vi "Convert to GEV Mono12Packed.vi"(10 "Source Image In":u8[](array[numeric])) -> (2 "Source Image Out":u8[](array[numeric]))   [LabVIEW 2021, in "DecodetoImage.lvlib"]
uses:
  DecodetoImage.lvlib
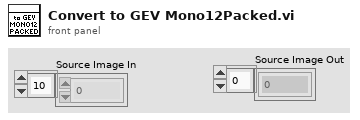
[diagram p1: front panel]
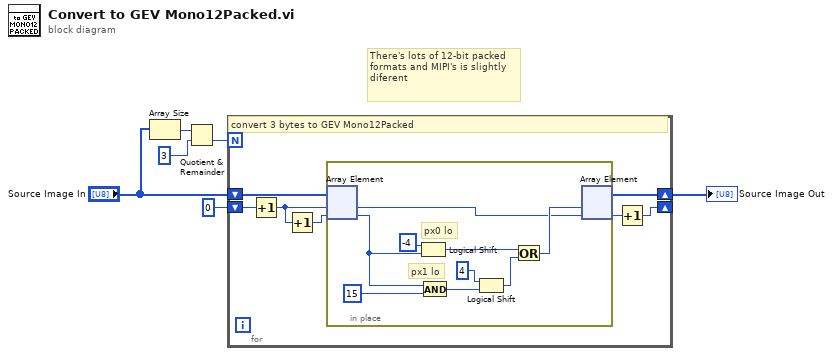
[diagram p0: block diagram]
diagram:
  # "There's lots of 12-bit packed formats and MIPI's is slightly diferent"
  n1 = Array Size(array="Source Image In") -> (size(s)=w4:i32)
  n2 = Quotient & Remainder(x=w4, y=3) -> (floor(x/y)=w6:i32)  [unwired: 1 out]
  n3 = for {
    N: w6 -> [_]
    shift-right: [w12] -> w2
    shift-left: "Source Image In" -> [w13]
    shift-right: [w7] -> _
    shift-left: 0 ("y") -> [w9]
    # "convert 3 bytes to GEV Mono12Packed"
    n4 = Increment(x=w9) -> (x+1=w11:i32)
    n5 = Increment(x=w11) -> (x+1=w10:i32)
    n6 = in-place {
      # "px0 lo"
      # "px1 lo"
      n7 = in-place-array #1(w13, w11, w10) -> (w14:u8, w15:u8)
      n8 = Logical Shift(y=i8 -4 ("x"), x=w15) -> (x << y=w17:u8)
      n9 = And(x=w15, y=u8 15) -> (x .and. y?=w20:u8)
      n10 = Logical Shift(y=i16 4, x=w20) -> (x << y=w18:u8)
      n11 = Or(x=w17, y=w18) -> (x .or. y?=w16:u8)
      n12 = in-place-array #1(w16, w14) -> (w12:u8[], w8:i32)  [unwired: 1 out]
    }
    n13 = Increment(x=w8) -> (x+1=w7:i32)
  }
  "Source Image Out" <- w2
